vi "Choose Connection.vi"(1 "STM connections":T1[](array[typedef])) -> (0 "Connection Ref":T1)   [LabVIEW 2019, in "RemoteControl.STM.lvclass"]
uses:
  RemoteControl.STM.lvclass
  <vilib>/NI/STM/TCP/TCP Connection Info.ctl
  <vilib>/NI/STM/SubVIs/MetaDataElement.ctl
  <vilib>/NI/STM/NI STM.lvlib
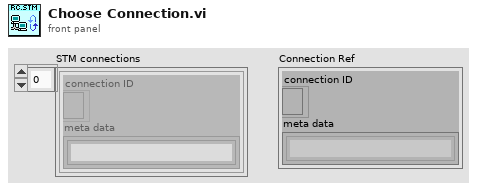
[diagram p1: front panel]
types:
  T1 = typedef "NI STM.lvlib/TCP Connection Info.ctl" = cluster{"connection ID":refnum<k5>, "meta data":T2[]}
  T2 = typedef "NI STM.lvlib/MetaDataElement.ctl" = string
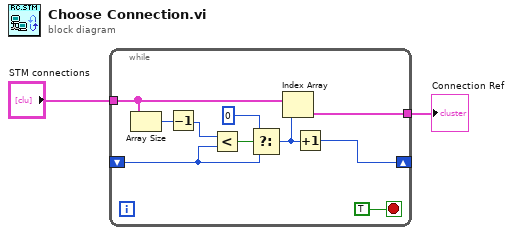
[diagram p0: block diagram]
diagram:
  n1 = while {
    tunnel: "STM connections" -> [w10]
    tunnel: [w12] -> w1
    shift-right: [w5] -> _
    shift-left: _ -> [w4]
    stop <- TRUE stop-if-true
    n2 = Array Size(array=w10) -> (size(s)=w9:i32)
    n3 = Decrement(x=w9) -> (x-1=w8:i32)
    n4 = Less?(x=w8, y=w4) -> (x < y?=w7:bool)
    n5 = Select(t=0 ("x-1"), s=w7, f=w4) -> (s? t:f=w3:i32)
    n6 = Index Array(array=w10, index=w3) -> (element=w12:T1)
    n7 = Increment(x=w3) -> (x+1=w5:i32)
  }
  "Connection Ref" <- w1
